vi "LVClass_DataClient GetDataNamesAndTypes.vi"(0 "DataClient in":refnum<class "DataClient.lvclass">, 11 "error in (no error)":errorcluster) -> (4 "DataClient out":refnum<class "DataClient.lvclass">, 6 "ArrayOfDataID":T1[](array[typedef]), 15 "error out":errorcluster)   [LabVIEW 2020, in "DataClient.lvclass"]
doc: "Slopes getter.\n\n--------------------------------------------------------------------------------\n\n<B>clientIn </B> : Client object.\n<B>clientOut </B> : Client object.\n<B>hasoslopes </B> : HasoSlopes object.\n<B>ErrorIn </B> : Error\n<B>ErrorOut </B> : Error\n\n--------------------------------------------------------------------------------"
uses:
  DataClient.lvclass
  ClientServerDataID.ctl
  ClientServerDataType.ctl
  DataClient.lvclass/DataClient.ctl
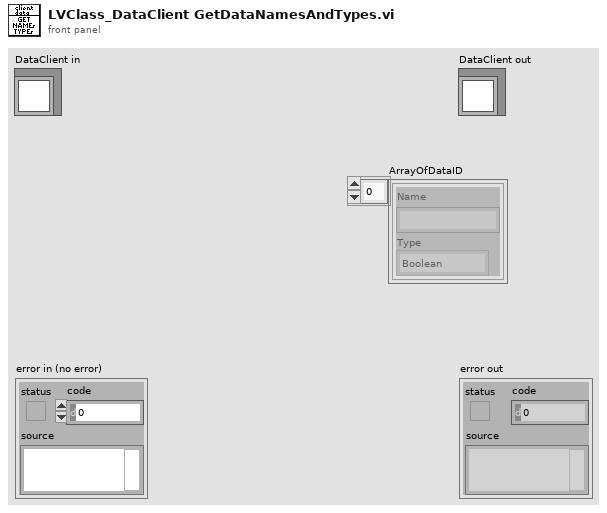
[diagram p1: front panel]
types:
  T1 = typedef "ClientServerDataID.ctl" = cluster{"Name":string, "Type":T2}
  T2 = typedef "ClientServerDataType.ctl" = enum16{"Boolean", "Integer", "Float", "String", "HasoSlopes", "Image"}
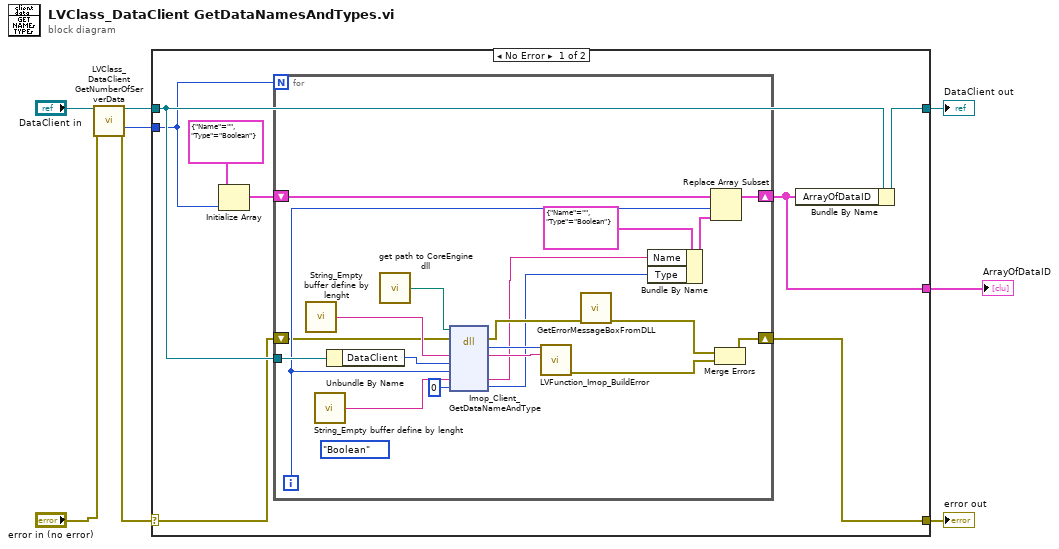
[diagram p0: block diagram]
diagram:
  n1 = call "LVClass_DataClient GetNumberOfServerData.vi"("DataClient in"="DataClient in", "error in (no error)"="error in (no error)") -> ("DataClient out"=w5:refnum<class "DataClient.lvclass">, "Number of data"=w2:i32, "error out"=w3:errorcluster)  [unwired: 11 in]
  n2 = case shown="No Error" w3 {
    selector: w3 -> [w10 w38]
    tunnel: [w9 w38] -> w8
    tunnel: [w15 w37] -> w7
    tunnel: w5 -> [w16 w37]
    tunnel: w2 -> [w11 _]
    tunnel: [w14 _] -> w1
    frame No Error {
      n3 = Initialize Array(T1 {"Name"="", "Type"=enum."Boolean"} ("DataID"), w11) -> (w12:T1[])
      n4 = for {
        N: w11 -> [_]
        tunnel: w16 -> [w26]
        shift-right: [w22] -> w14
        shift-left: w12 -> [w24]
        shift-right: [w17] -> w9
        shift-left: w10 -> [w18]
        i -> [w23]
        (unwired) ClientServerDataType."Boolean" ("Type")
        n5 = call "String_Empty buffer define by lenght.vi"() -> ("Empty buffer"=w34:string)  [unwired: 1 in]
        n6 = call "String_Empty buffer define by lenght.vi"() -> ("Empty buffer"=w20:string)  [unwired: 1 in]
        n7 = Unbundle By Name(w26) -> ("DataClient"=w31:i32)
        n8 = call "get path to CoreEngine dll.vi"() -> ("path to c_interface_vc100.dll"=w33:path)  [unwired: 12 in, 3 out]
        n9 = dll-call lib="D:/soft/HASO_v3/SVN_trunk/ImOpCoreEngine4_LV2011/DLLs/c_interface_vc100.dll" fn="Imop_Client_GetDataNameAndType"(path in=w33, error in=w18, "message"=w34, "client"=w31, "index"=w23, "data_name"=w20, "data_type"=0) -> (error out=w32:errorcluster, "return type"=w36:i32, "message"=w35:string, "data_name"=w28:string, "data_type"=w27:i32)  [unwired: 3 in, 1 out]
        n10 = call "LVFunction_Imop_BuildError.vi"("code"=w36, "String to Prepend to source (\"\")"=w35) -> ("error out"=w29:errorcluster)  [unwired: 13 in]
        n11 = call "GetErrorMessageBoxFromDLL.vi"("error IN"=w32) -> ("error OUT"=w30:errorcluster)  [unwired: 10 in]
        n12 = Bundle By Name(cluster=T1 {"Name"="", "Type"=enum."Boolean"} ("DataID"), "Name"=w28, "Type"=w27) -> (w21:T1)
        n13 = Replace Array Subset(array=w24, new element=w21, index=w23) -> (w22:T1[])
        n14 = Merge Errors(w30, w29) -> (w17:errorcluster)
      }
      n15 = Bundle By Name(cluster=w16, "ArrayOfDataID"=w14) -> (w15:refnum<class "DataClient.lvclass">)
    }
    frame Error {
    }
  }
  "error out" <- w8
  "DataClient out" <- w7
  "ArrayOfDataID" <- w1
